vi "未命名 2.vi"() -> ()   [LabVIEW 2012]
panel:
  out "结果字符串":string
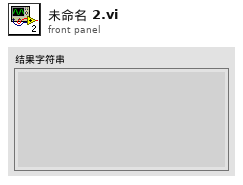
[diagram p1: front panel]
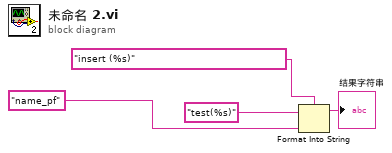
[diagram p0: block diagram]
diagram:
  n1 = Format Into String(format string="insert (%s)" ("格式字符串"), initial string="test(%s)" ("字符串"), "name_pf" ("输入 1")) -> (resulting string=→"结果字符串":string)  [unwired: 1 in, 1 out]
